vi "AlliGator Save Multiple ROIs v3.vi"(8 "Error In":errorcluster, 9 "Default File Name":string="Multiple ROIs.roiN", 10 "Destination Folder (Default: last)":path=path "", 11 "ROI Description":T1 {"Named ROI Descriptions"."ROI Descriptor"."Contours"."Type" items=["No Selection", "Point", "Line", "Rectangle", "Oval", "Polygon", "Freehand Region", "Annulus", "Unused2", "Unused3", "Broken Line", "Freehand Line", "Rotated Rectangle"]}) -> (0 "Error Out":errorcluster, 3 "Notebook Message":string)   [LabVIEW 2021, in "AlliGator ROIs.lvlib"]
doc: "Save multiple ROIs."
uses:
  AlliGator ROIs.lvlib
  Image/Image Control Multiple ROIs Description v2.ctl
  Image/Named ROI Description.ctl
  2f6536f2-4c73-4be5-9a90-4bb6a5b7d0f4.vi
  <vilib>/JDP Science/JSONtext/Variant to JSON Text.vi
  <vilib>/JDP Science/JSONtext/LVClass Serializer/JSONtext LVClass Serializer.lvclass
  Image/Image.lvlib
panel:
  # "see the AlliGator License on the block diagram (Ctrl+E or Window:Show Block Diagram)"
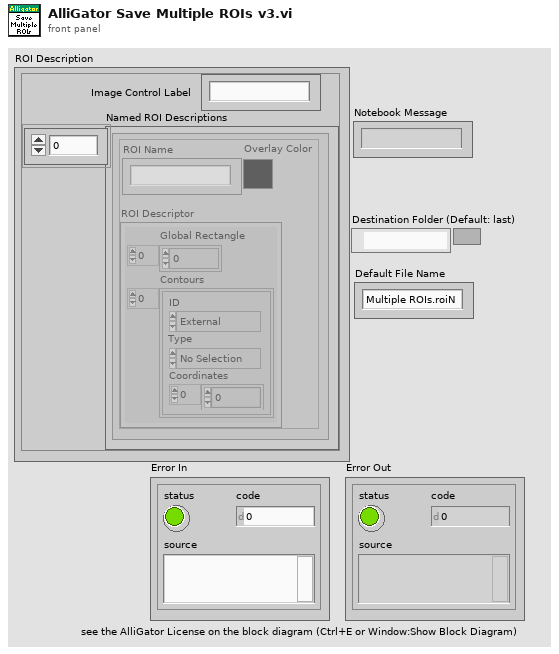
[diagram p1: front panel]
types:
  T1 = typedef "Image.lvlib/Image Control Multiple ROIs Description v2.ctl" = cluster{"Image Control Label":string, "Named ROI Descriptions":T2[]}
  T2 = typedef "Image.lvlib/Named ROI Description.ctl" = cluster{"ROI Descriptor":T3, "ROI Name":string, "Overlay Color":u32}
  T3 = typedef "ROI Descriptor" = cluster{"Global Rectangle":i32[], "Contours":cluster{"ID":enum32{"External", "Internal"}, "Type":u32, "Coordinates":i32[]}[]}
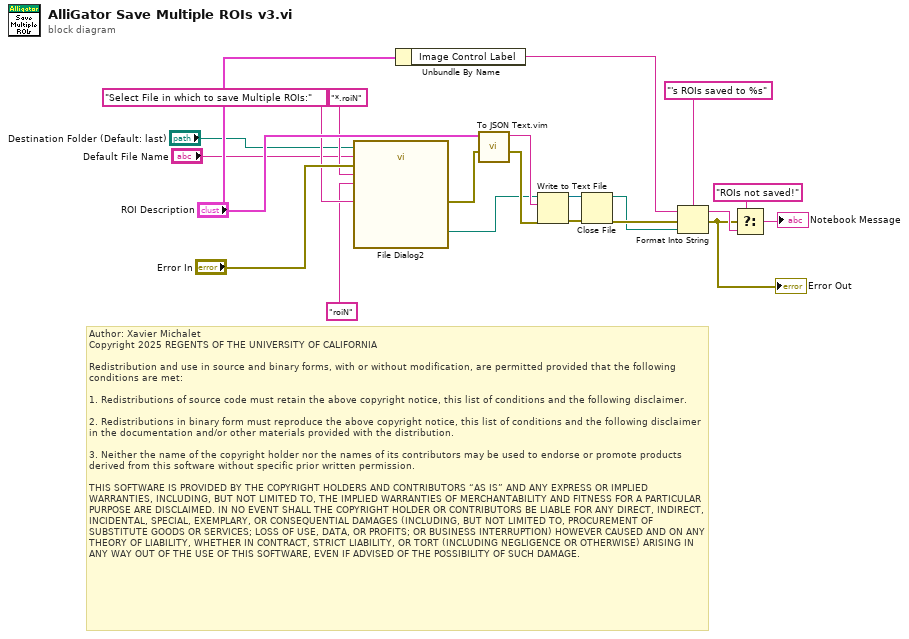
[diagram p0: block diagram]
diagram:
  # "Author: Xavier Michalet\nCopyright 2025 REGENTS OF THE UNIVERSITY OF CALIFORNIA\n\nRedistribution and use in source and binary forms, with or without modification, are permitted provided that the following conditions are met:\n\n1. Redistributions of source code must retain the above copyright notice, this list of conditions and the following disclaimer.\n\n2. Redistributions in binary form must reproduce the above copyright notice, this list of conditions and the following disclaimer in the documentation and/or other materials provided with the distribution.\n\n3. Neither the name of the copyright holder nor the names of its contributors may be used to endorse or promote products derived from this software without specific prior written permission.\n\nTHIS SOFTWARE IS PROVIDED BY THE COPYRIGHT HOLDERS AND CONTRIBUTORS “AS IS” AND ANY EXPRESS OR IMPLIED WARRANTIES, INCLUDING, BUT NOT LIMITED TO, THE IMPLIED WARRANTIES OF MERCHANTABILITY AND FITNESS FOR A PARTICULAR PURPOSE ARE DISCLAIMED. IN NO EVENT SHALL THE COPYRIGHT HOLDER OR CONTRIBUTORS BE LIABLE FOR ANY DIRECT, INDIRECT, INCIDENTAL, SPECIAL, EXEMPLARY, OR CONSEQUENTIAL DAMAGES (INCLUDING, BUT NOT LIMITED TO, PROCUREMENT OF SUBSTITUTE GOODS OR SERVICES; LOSS OF USE, DATA, OR PROFITS; OR BUSINESS INTERRUPTION) HOWEVER CAUSED AND ON ANY THEORY OF LIABILITY, WHETHER IN CONTRACT, STRICT LIABILITY, OR TORT (INCLUDING NEGLIGENCE OR OTHERWISE) ARISING IN ANY WAY OUT OF THE USE OF THIS SOFTWARE, EVEN IF ADVISED OF THE POSSIBILITY OF SUCH DAMAGE."
  n1 = call "File Dialog2"("start path"="Destination Folder (Default: last)", "prompt"="Select File in which to save Multiple ROIs:" ("Prompt"), "default name"="Default File Name", "error in"="Error In", "pattern (all files)"="*.roiN" ("Pattern (*.xml;*.XML)"), "pattern label"="roiN" ("File Extension (xml)")) -> ("selected path"=w2:path, "error out"=w3:errorcluster)  [unwired: 6 in, 2 out]
  n2 = Unbundle By Name("ROI Description") -> ("Image Control Label"=w15:string)
  n3 = call "To JSON Text.vim"("error in (no error)"=w3, "Anything"="ROI Description") -> ("error out"=w4:errorcluster, "<JSON>"=w6:string)  [unwired: 8 in]
  n4 = Write to Text File(file (use dialog)=w2, text=w6, error in=w4) -> (refnum out=w7:refnum<file>, error out=w5:errorcluster)  [unwired: 1 in, 1 out]
  n5 = Close File(refnum=w7, error in=w5) -> (path=w17:path, error out=w18:errorcluster)
  n6 = Format Into String(format string="'s ROIs saved to %s", initial string=w15, error in=w18, w17) -> (resulting string=w19:string, error out=w12:errorcluster)
  "Error Out" <- w12
  n7 = Select(t="ROIs not saved!", s=w12, f=w19) -> (s? t:f=→"Notebook Message":string)
